vi "DMM_Initialize.vi"(2 "Comments":string, 3 "Baseline Pick":enum16{"Manual", "Auto"}(ring), 4 "File Path":path, 5 "Sampling Rate (point / sec)":u32, 6 "Measurement":enum16{"Resistance", "Current"}(ring), 7 "DMM Serial Port":refnum<visa-resource-name>) -> (0 "State":string="Initialize", 1 "Output DMMP":refnum<class "DMMP.lvclass">)   [LabVIEW 2014]
uses:
  DMMP.lvclass
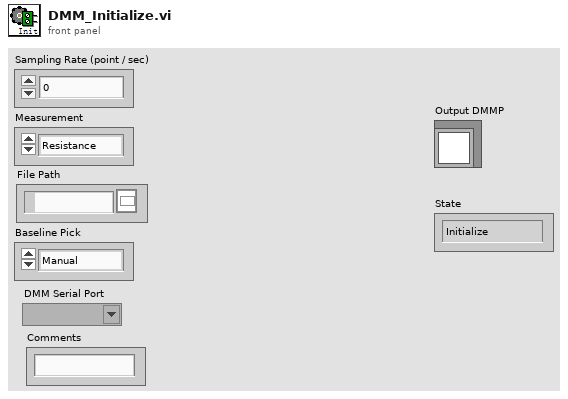
[diagram p1: front panel]
types:
  T1 = cluster{"Sampling Rate (point / sec)":u32, "Measurement":enum16{"Resistance", "Current"}, "DMM Serial Port":refnum<visa-resource-name>, "File Path":path, "Baseline Pick":enum16{"Manual", "Auto"}, "Comments":string}
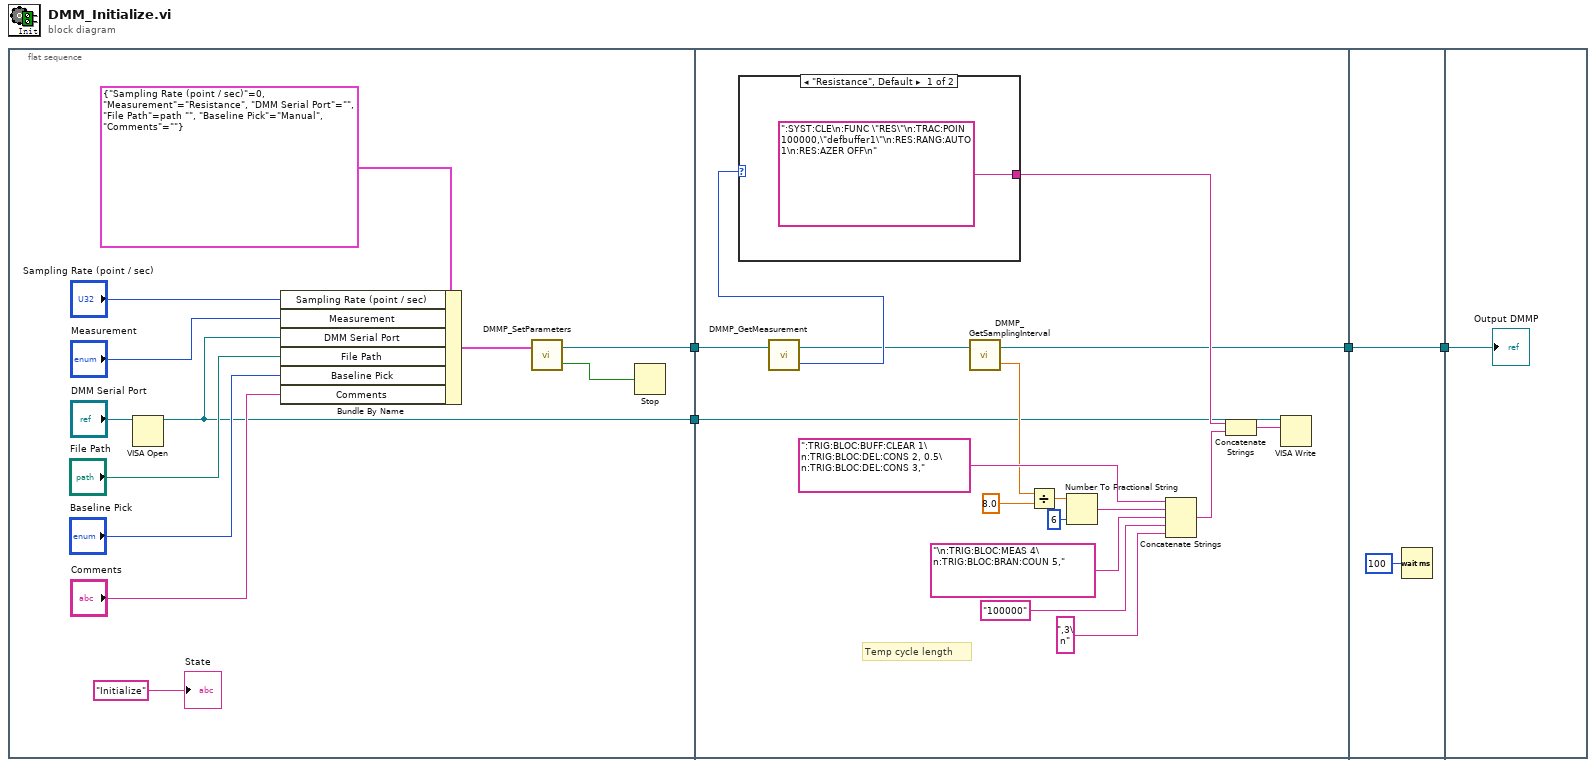
[diagram p0: block diagram]
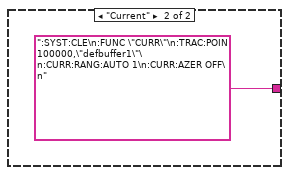
[diagram p2: hidden frame]
diagram:
  n1 = flat-sequence {
    tunnel: [w9] -> w4
    tunnel: [w5] -> w1
    tunnel: w4 -> [w33]
    tunnel: [w18] -> w3
    tunnel: w1 -> [w17]
    tunnel: w3 -> [w37]
    tunnel: [w37] -> w2
    tunnel: w2 -> [w38]
    frame #0 {
      n2 = VISA Open(VISA resource name="DMM Serial Port") -> (VISA resource name=w5:refnum<visa-resource-name>)  [unwired: 4 in, 1 out]
      n3 = Bundle By Name(cluster=T1 {"Sampling Rate (point / sec)"=0, "Measurement"=enum."Resistance", "DMM Serial Port"="", "File Path"=path "", "Baseline Pick"=enum."Manual", "Comments"=""}, "Sampling Rate (point / sec)"="Sampling Rate (point / sec)", "Measurement"="Measurement", "DMM Serial Port"=w5, "File Path"="File Path", "Baseline Pick"="Baseline Pick", "Comments"="Comments") -> (w10:T1)
      n4 = call "DMMP_SetParameters.vi"("Input Parameters"=w10) -> ("Error?"=w8:bool, "DMMP.lvclass"=w9:refnum<class "DMMP.lvclass">)  [unwired: 1 in]
      n5 = Stop(stop? (T)=w8) -> ()
      "State" <- "Initialize"
    }
    frame #1 {
      # "Temp cycle length"
      n6 = call "DMMP_GetMeasurement.vi"("Input DMMP"=w33) -> ("Measurement"=w32:enum16{"Resistance", "Current"}, "Output DMMP"=w20:refnum<class "DMMP.lvclass">)  [unwired: 1 in]
      n7 = case shown="\"Resistance\", Default" w32 {
        tunnel: [":SYST:CLE\n:FUNC \"RES\"\n:TRAC:POIN 100000,\"defbuffer1\"\n:RES:RANG:AUTO 1\n:RES:AZER OFF\n" ("write buffer") ":SYST:CLE\n:FUNC \"CURR\"\n:TRAC:POIN 100000,\"defbuffer1\"\n:CURR:RANG:AUTO 1\n:CURR:AZER OFF\n" ("write buffer")] -> w31
        frame "Resistance", Default {
        }
        frame "Current" {
        }
      }
      n8 = call "DMMP_GetSamplingInterval.vi"("Input DMMP"=w20) -> ("Sampling Interval (ms)"=w19:dbl, "Output DMMP"=w18:refnum<class "DMMP.lvclass">)  [unwired: 1 in]
      n9 = Divide(x=w19, y=8.0) -> (x/y=w22:dbl)
      n10 = Number To Fractional String(number=w22, precision (6)=i16 6) -> (F-format string=w27:string)  [unwired: 2 in]
      n11 = Concatenate Strings(":TRIG:BLOC:BUFF:CLEAR 1\n:TRIG:BLOC:DEL:CONS 2, 0.5\n:TRIG:BLOC:DEL:CONS 3,", w27, "\n:TRIG:BLOC:MEAS 4\n:TRIG:BLOC:BRAN:COUN 5," ("string"), "100000" ("string"), ",3\n" ("string")) -> (w21:string)
      n12 = Concatenate Strings(w31, w21) -> (w30:string)
      n13 = VISA Write(VISA resource name=w17, write buffer=w30) -> ()  [unwired: 1 in, 3 out]
    }
    frame #2 {
      n14 = Wait (ms)(milliseconds to wait=u32 100) -> ()  [unwired: 1 out]
    }
    frame #3 {
      "Output DMMP" <- w38
    }
  }
